vi "OPA.GetShutterState.vi"(8 "error in (no error)":errorcluster, 11 "OPA in":refnum<class "OPA.lvclass">) -> (0 "error out":errorcluster, 2 "Shutter State":bool, 3 "OPA out":refnum<class "OPA.lvclass">)   [LabVIEW 2019, in "OPA.lvclass"]
uses:
  OPA.lvclass
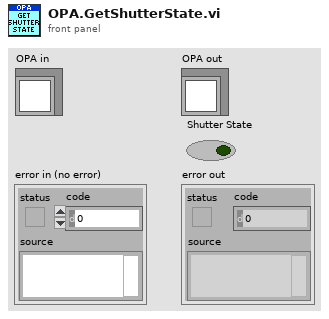
[diagram p1: front panel]
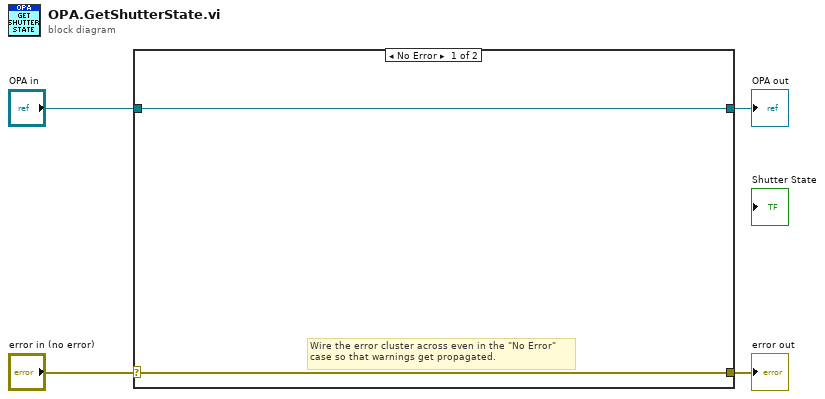
[diagram p0: block diagram]
diagram:
  n1 = case shown="No Error" "error in (no error)" {
    selector: "error in (no error)" -> [w5 w8]
    tunnel: [w5 w8] -> w3
    tunnel: [w6 w7] -> w1
    tunnel: "OPA in" -> [w6 w7]
    frame No Error {
      # "Wire the error cluster across even in the \"No Error\"\ncase so that warnings get propagated."
    }
    frame Error {
    }
  }
  "error out" <- w3
  "OPA out" <- w1
